vi "UI_Template_Add.vi"() -> ()   [LabVIEW 2014]
uses:
  Terminal_Global_User_name.vi
panel:
  in  "退出":bool
  in  "添加模板":bool
  in  "添加载荷谱模板":string[][](table)
  in  "请输入模板名称":string
  # "增加载荷谱模板"
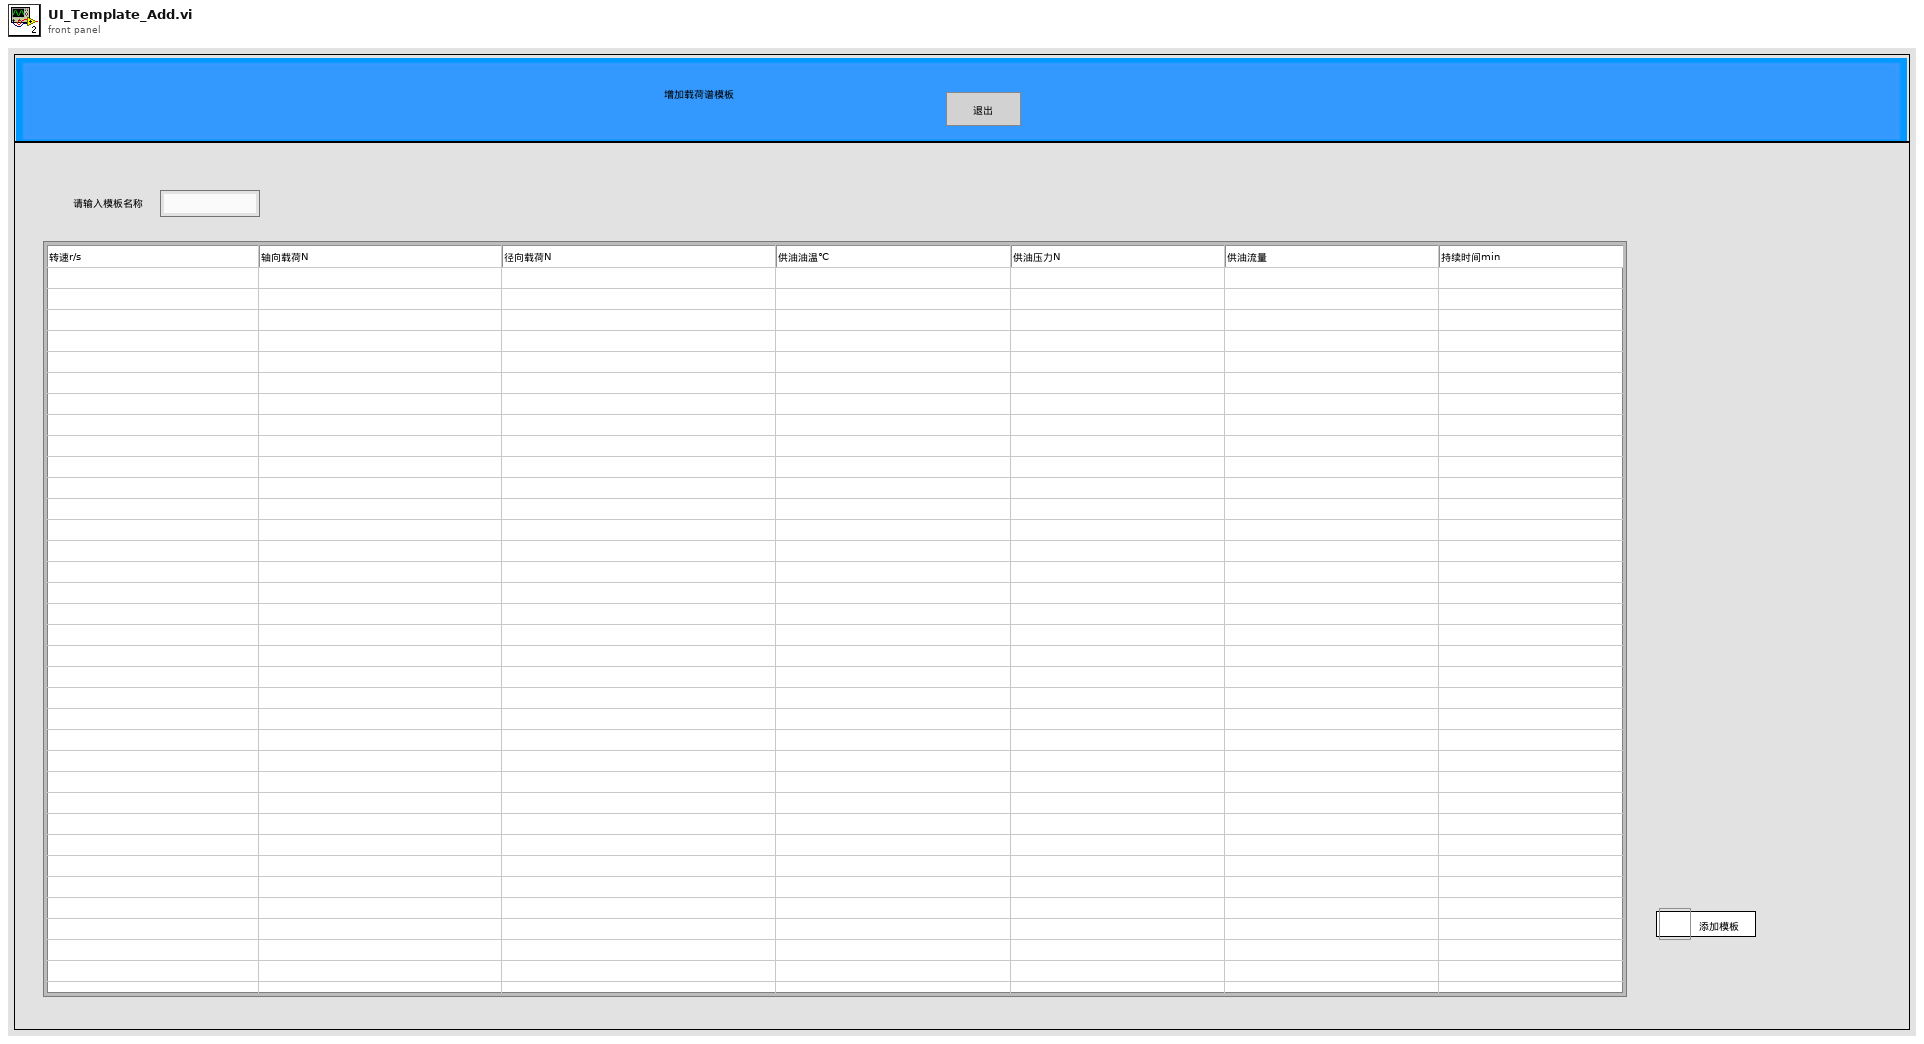
[diagram p1: front panel]
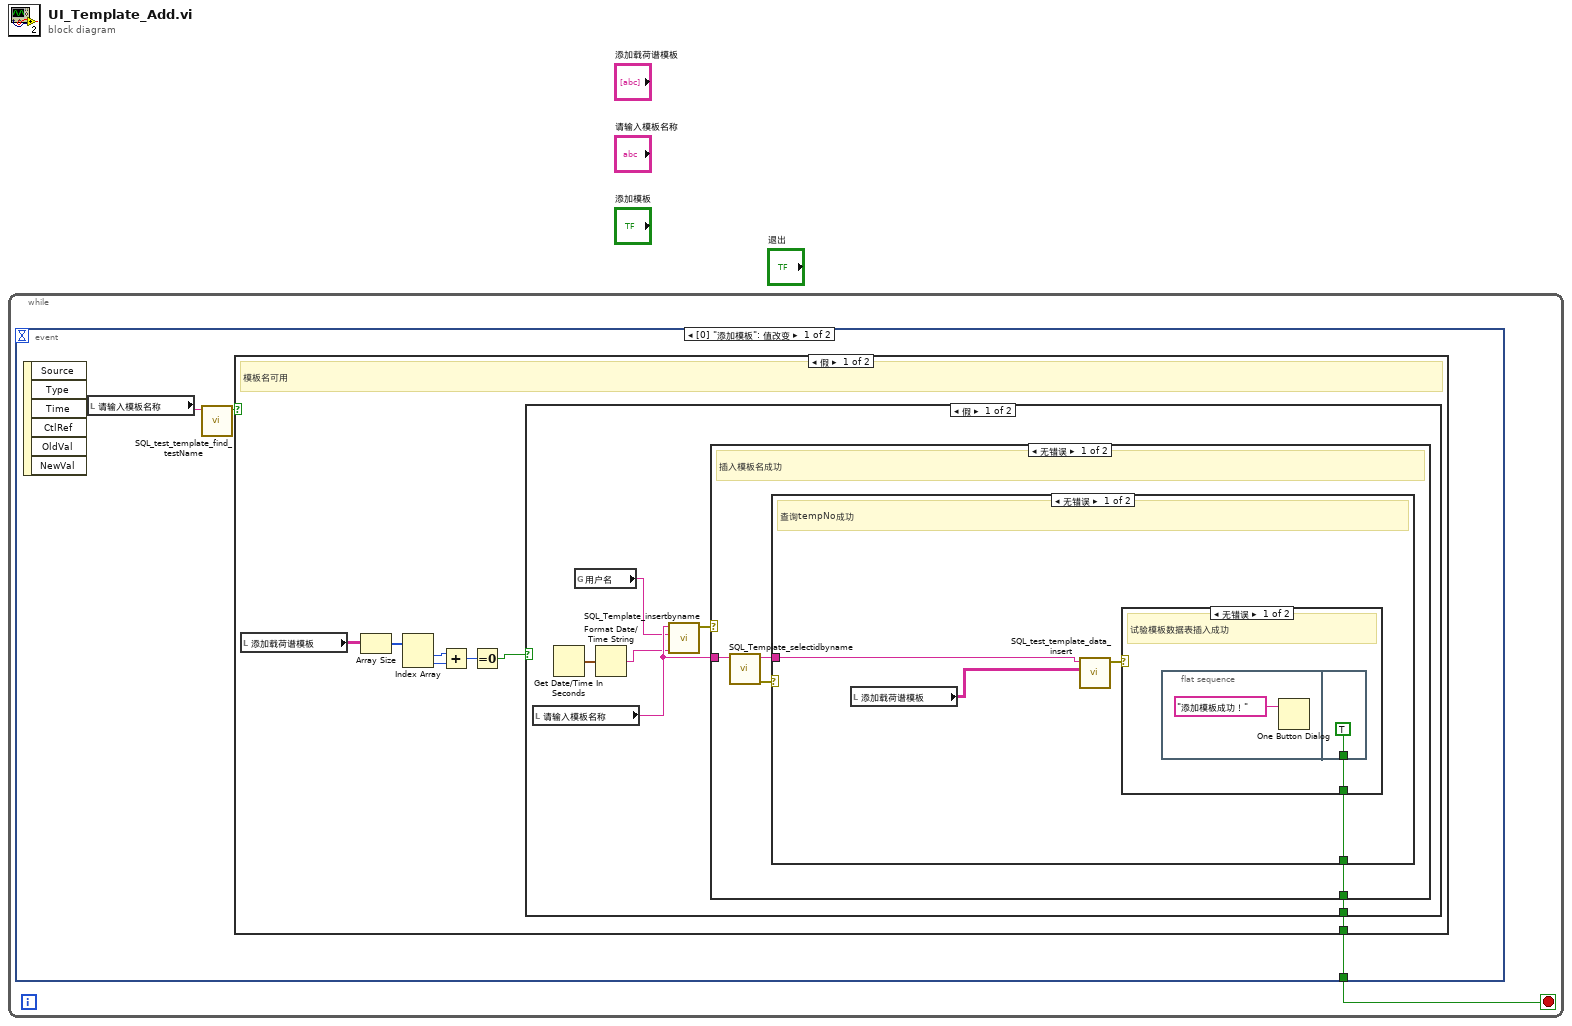
[diagram p0: block diagram]
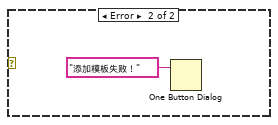
[diagram p2: hidden frame]
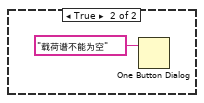
[diagram p5: hidden frame]
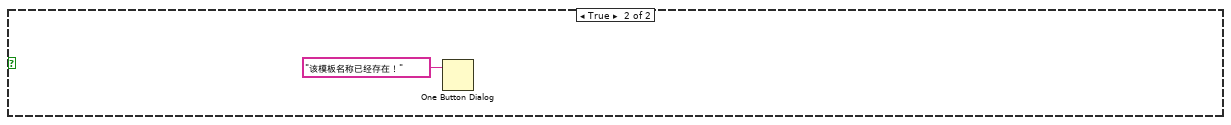
[diagram p6: hidden frame]
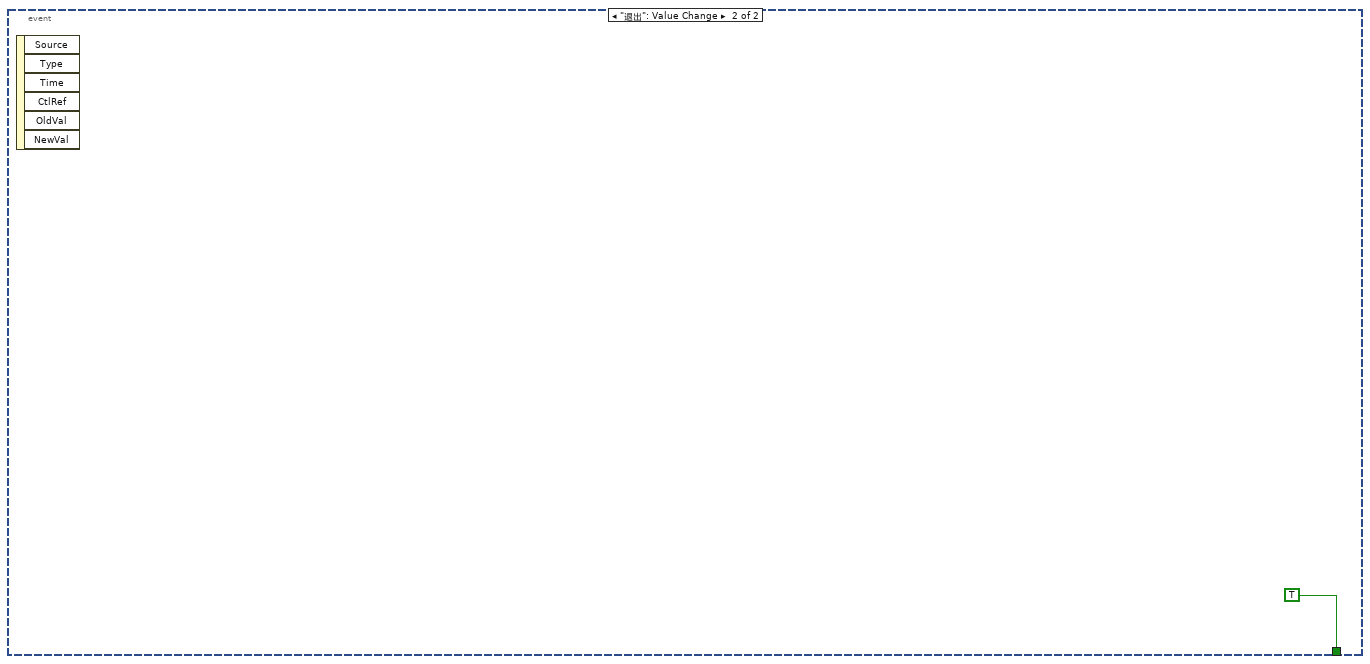
[diagram p7: hidden frame]
diagram:
  n1 = while {
    stop <- w1 stop-if-true
    n2 = event shown="[0] \"添加模板\": 值改变" {
      selector: _ -> [_ _]
      dyn-events: _ -> [_ _]
      timeout: _ -> [_ _]
      tunnel: [w2 TRUE] -> w1
      event "添加模板": Value Change {
        n3 = event-data() -> ()  [unwired: 1 in, 6 out]
        n4 = local read "请输入模板名称"() -> (w3:string)
        n5 = call "SQL_test_template_find_testName.vi"("模板名称"=w3) -> ("模板是否存在"=w4:bool)  [unwired: 10 in]
        n6 = case shown="假" w4 {
          tunnel: [w11 _] -> w2
          frame False {
            # "模板名可用"
            n7 = local read "添加载荷谱模板"() -> (w10:string[][])
            n8 = Array Size(array=w10) -> (size(s)=w7:i32[])
            n9 = Index Array(array=w7) -> (element #1=w8:i32, element #2=w9:i32)  [unwired: 2 in]
            n10 = Add(x=w8, y=w9) -> (x+y=w6:i32)
            n11 = Equal To 0?(x=w6) -> (x = 0?=w5:bool)
            n12 = case shown="假" w5 {
              tunnel: [w15 _] -> w11
              frame False {
                n13 = local read "请输入模板名称"() -> (w17:string)
                n14 = Get Date/Time In Seconds() -> (seconds since 1Jan1904=w13:timestamp)
                n15 = global read "Terminal_Global_User_name.vi" "用户名"() -> (w14:string)
                n16 = Format Date/Time String(seconds (now)=w13) -> (date/time string=w12:string)  [unwired: 2 in]
                n17 = call "SQL_Template_insertbyname.vi"("创建时间"=w12, "创建人"=w14, "tempName"=w17) -> ("error out"=w16:errorcluster)  [unwired: 8 in]
                n18 = case shown="无错误" w16 {
                  tunnel: w17 -> [w21 _]
                  tunnel: [w18 _] -> w15
                  frame No Error {
                    # "插入模板名成功"
                    n19 = call "SQL_Template_selectidbyname.vi"("模板名称"=w21) -> ("error out"=w20:errorcluster, "tempNo"=w19:string)  [unwired: 9 in]
                    n20 = case shown="无错误" w20 {
                      tunnel: w19 -> [w25 _]
                      tunnel: [w24 _] -> w18
                      frame No Error {
                        # "查询tempNo成功"
                        n21 = local read "添加载荷谱模板"() -> (w22:string[][])
                        n22 = call "SQL_test_template_data_insert.vi"("表格控件"=w22, "tempNo"=w25) -> ("error out"=w23:errorcluster)  [unwired: 9 in]
                        n23 = case shown="无错误" w23 {
                          tunnel: [w26 _] -> w24
                          frame No Error {
                            # "试验模板数据表插入成功"
                            n24 = flat-sequence {
                              tunnel: [TRUE] -> w26
                              frame #0 {
                                n25 = One Button Dialog(message="添加模板成功！" ("消息")) -> ()  [unwired: 1 in, 1 out]
                              }
                              frame #1 {
                              }
                            }
                          }
                          frame Error {
                            n26 = One Button Dialog(message="添加模板失败！" ("消息")) -> ()  [unwired: 1 in, 1 out]
                          }
                        }
                      }
                      frame Error {
                      }
                    }
                  }
                  frame Error {
                  }
                }
              }
              frame True {
                n27 = One Button Dialog(message="载荷谱不能为空" ("消息")) -> ()  [unwired: 1 in, 1 out]
              }
            }
          }
          frame True {
            n28 = One Button Dialog(message="该模板名称已经存在！" ("消息")) -> ()  [unwired: 1 in, 1 out]
          }
        }
      }
      event "退出": Value Change {
        n29 = event-data() -> ()  [unwired: 1 in, 6 out]
      }
    }
  }
